vi "filterWheelThorlabsGetPosition.vi"() -> (0 "port":i32, 1 "read buffer":string)   [LabVIEW 2017]
uses:
  globalDevices.vi
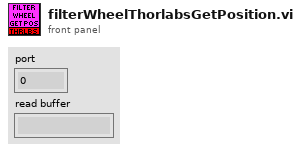
[diagram p1: front panel]
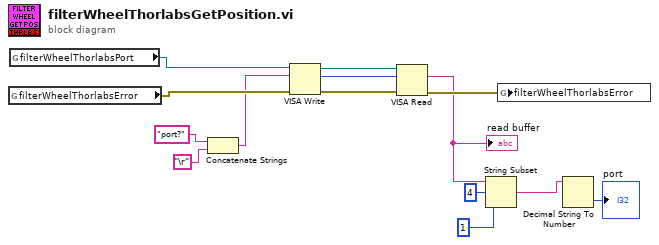
[diagram p0: block diagram]
diagram:
  n1 = global read "globalDevices.vi" "filterWheelThorlabsError"() -> (w13:errorcluster)
  n2 = global read "globalDevices.vi" "filterWheelThorlabsPort"() -> (w14:refnum<visa-resource-name>)
  n3 = Concatenate Strings("port?" ("write buffer"), "\r") -> (w5:string)
  n4 = VISA Write(VISA resource name=w14, write buffer=w5, error in (no error)=w13) -> (VISA resource name out=w12:refnum<visa-resource-name>, return count=w11:u32, error out=w10:errorcluster)
  n5 = VISA Read(VISA resource name=w12, byte count=w11, error in (no error)=w10) -> (read buffer=w4:string, error out=w9:errorcluster)  [unwired: 2 out]
  "read buffer" <- w4
  n6 = String Subset(string=w4, offset (0)=4, length (rest)=1 ("length (rest)")) -> (substring=w1:string)
  n7 = global write "globalDevices.vi" "filterWheelThorlabsError"(w9) -> ()
  n8 = Decimal String To Number(string=w1) -> (number=→"port":i32)  [unwired: 2 in, 1 out]
